vi "location_x.vi"() -> ()   [LabVIEW 2018]
panel:
  in  "当前位置-X":dbl
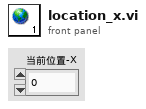
[diagram p1: front panel]
diagram:
